vi "Start-values.vi"(8 "error in":errorcluster, 11 "UI ref. in":refnum<data-value>) -> (0 "error IO":errorcluster, 3 "UI ref.":refnum<data-value>)   [LabVIEW 2013, in "CameraVision.lvlib" / "CV-UI.lvclass"]
doc: "This function sets appropriate acquisition values for the GUI buttons and selectors. Currently only the value of the image refresh button is changed to true (with event signalling), to enable the continuous update of the displays during acquisition."
uses:
  CV-UI.lvclass
  CV-UI.lvclass/CV-UI.ctl
  Read Control refs.vi
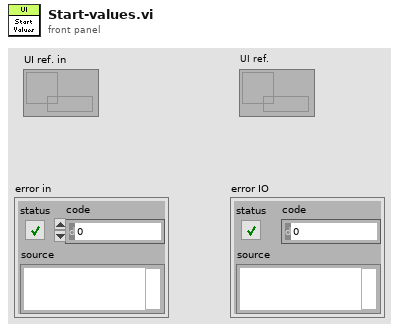
[diagram p1: front panel]
types:
  T1 = typedef "CameraVision.lvlib/CV-UI.lvclass/Control-names.ctl" = enum16{"Start acquisition", "Activate", "Stop acquisition", "Settings type", "Load settings", "Save settings", "Import images", "Camera selector", "Image type selector", "Batch browser", "Image refresh", "Parameter tabs", "Displays", "Processing tabs", "Processing selector", "Map characteristic", "Show info", "Manual trigger"}
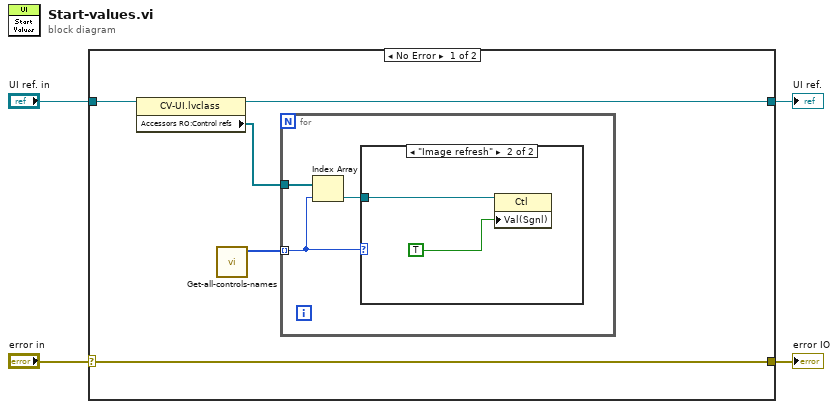
[diagram p0: block diagram]
diagram:
  n1 = case shown="No Error" "error in" {
    selector: "error in" -> [w9 w16]
    tunnel: "UI ref. in" -> [w6 w15]
    tunnel: [w9 w16] -> w4
    tunnel: [w5 w15] -> w1
    frame No Error {
      n2 = property class="CV-UI.lvclass"(reference=w6) -> (reference out=w5:refnum<data-value>, "Accessors RO:Control refs"=w7:refnum<vi>[])  [unwired: 1 in, 1 out]
      n3 = call "Get-all-controls-names.vi"() -> ("Controls"=w8:T1[])  [unwired: 11 in]
      n4 = for {
        tunnel: w8 -> [w10] mode=indexing
        tunnel: w7 -> [w12]
        n5 = Index Array(array=w12, index=w10) -> (element=w11:refnum<vi>)
        n6 = case shown="\"Image refresh\"" w10 {
          tunnel: w11 -> [_ w14]
          frame Default {
          }
          frame "Image refresh" {
            n7 = property class="Ctl"(reference=w14, "Val(Sgnl)"=TRUE) -> ()  [unwired: 1 in, 2 out]
          }
        }
      }
    }
    frame Error {
    }
  }
  "error IO" <- w4
  "UI ref." <- w1
